vi "Generator Lesson 4.vi"() -> ()   [LabVIEW 2024]
uses:
  <vilib>/Instr/_visa.llb/VISA Configure Serial Port (Instr).vi
panel:
  out "kW":dbl(knob) scale=0.0..1000.0
  in  "Load Level (0-1000)":dbl(slide) scale=0.0..1000.0
  in  "Motor Speed":dbl(slide) scale=0.0..255.0
  in  "stop":bool
  out "Waveform Chart":dbl(graph)
  in  "VISA resource name":refnum<visa-resource-name>
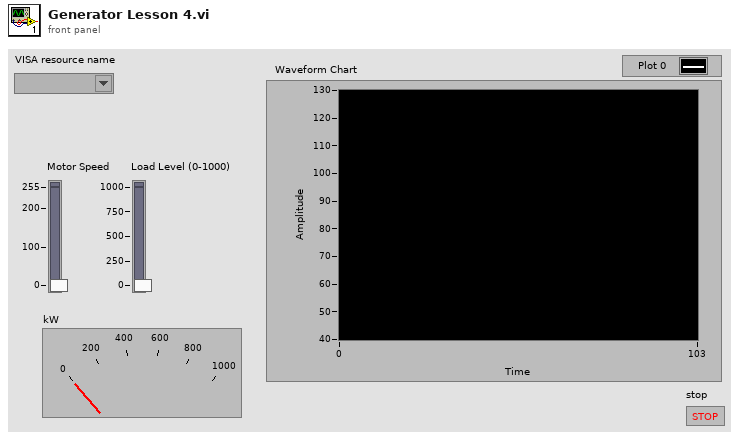
[diagram p1: front panel]
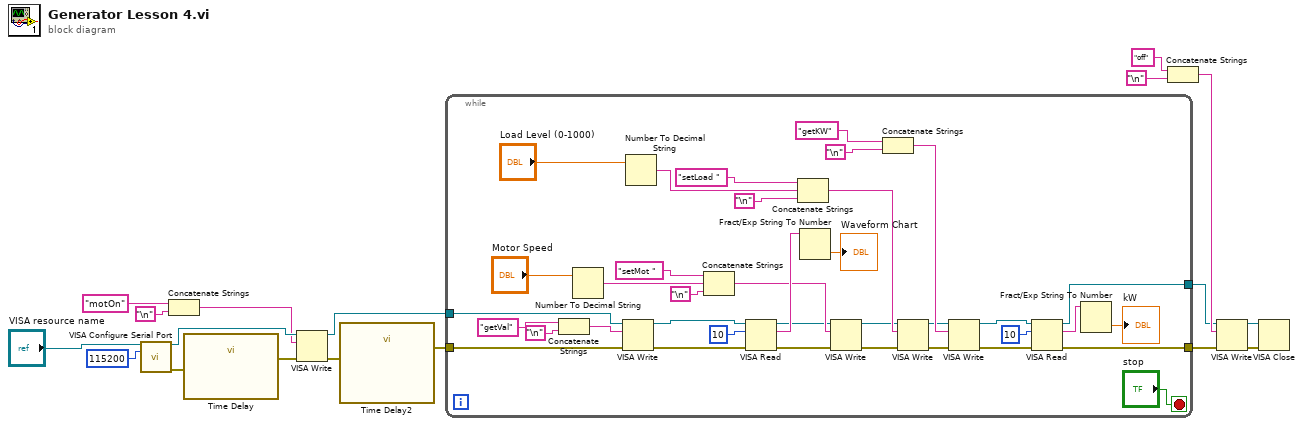
[diagram p0: block diagram]
diagram:
  n1 = call-poly "VISA Configure Serial Port"("VISA resource name"="VISA resource name", "baud rate (9600)"=u32 115200) -> ("VISA resource name out"=w15:refnum<visa-resource-name>, "error out"=w16:errorcluster)  [unwired: 12 in]
  n2 = Concatenate Strings("motOn", "\n") -> (w11:string)
  n3 = call "Time Delay"("error in (no error)"=w16) -> ("error out"=w14:errorcluster)  [unwired: 10 in]
  n4 = VISA Write(VISA resource name=w15, write buffer=w11, error in (no error)=w14) -> (VISA resource name out=w8:refnum<visa-resource-name>, error out=w10:errorcluster)  [unwired: 1 out]
  n5 = call "Time Delay2"("error in (no error)"=w10) -> ("error out"=w9:errorcluster)  [unwired: 10 in]
  n6 = while {
    tunnel: w9 -> [w53]
    tunnel: w8 -> [w52]
    tunnel: [w22] -> w4
    tunnel: [w21] -> w3
    stop <- "stop" stop-if-true
    n7 = Concatenate Strings("getVal", "\n") -> (w51:string)
    n8 = Number To Decimal String(number="Motor Speed") -> (decimal integer string=w38:string)  [unwired: 1 in]
    n9 = VISA Write(VISA resource name=w52, write buffer=w51, error in (no error)=w53) -> (VISA resource name out=w50:refnum<visa-resource-name>, error out=w49:errorcluster)  [unwired: 1 out]
    n10 = Number To Decimal String(number="Load Level (0-1000)") -> (decimal integer string=w34:string)  [unwired: 1 in]
    n11 = Concatenate Strings("setMot ", w38, "\n") -> (w42:string)
    n12 = VISA Read(VISA resource name=w50, byte count=u32 10, error in (no error)=w49) -> (VISA resource name out=w41:refnum<visa-resource-name>, read buffer=w47:string, error out=w40:errorcluster)  [unwired: 1 out]
    n13 = Concatenate Strings("setLoad ", w34, "\n") -> (w33:string)
    n14 = Fract/Exp String To Number(string=w47) -> (number=→"Waveform Chart":dbl)  [unwired: 3 in, 1 out]
    n15 = VISA Write(VISA resource name=w41, write buffer=w42, error in (no error)=w40) -> (VISA resource name out=w32:refnum<visa-resource-name>, error out=w31:errorcluster)  [unwired: 1 out]
    n16 = Concatenate Strings("getKW", "\n") -> (w28:string)
    n17 = VISA Write(VISA resource name=w32, write buffer=w33, error in (no error)=w31) -> (VISA resource name out=w24:refnum<visa-resource-name>, error out=w23:errorcluster)  [unwired: 1 out]
    n18 = VISA Write(VISA resource name=w24, write buffer=w28, error in (no error)=w23) -> (VISA resource name out=w27:refnum<visa-resource-name>, error out=w26:errorcluster)  [unwired: 1 out]
    n19 = VISA Read(VISA resource name=w27, byte count=u32 10, error in (no error)=w26) -> (VISA resource name out=w22:refnum<visa-resource-name>, read buffer=w20:string, error out=w21:errorcluster)  [unwired: 1 out]
    n20 = Fract/Exp String To Number(string=w20) -> (number=→"kW":dbl)  [unwired: 3 in, 1 out]
  }
  n21 = Concatenate Strings("off", "\n") -> (w5:string)
  n22 = VISA Write(VISA resource name=w4, write buffer=w5, error in (no error)=w3) -> (VISA resource name out=w2:refnum<visa-resource-name>, error out=w1:errorcluster)  [unwired: 1 out]
  n23 = VISA Close(VISA resource name=w2, error in (no error)=w1) -> ()  [unwired: 1 out]
